vi "Initialize Motor.vi"() -> ()   [LabVIEW 2010]
panel:
  in  "Control units?":bool
  out "Enable\nReturn Value":i16
  out "Program\nReturn Value":i16
  out "Init\nReturn\nValue":i16
  out "Open\nDriver\nReturn\nValue":i16
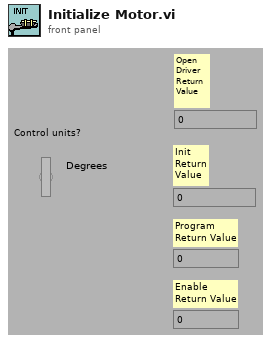
[diagram p1: front panel]
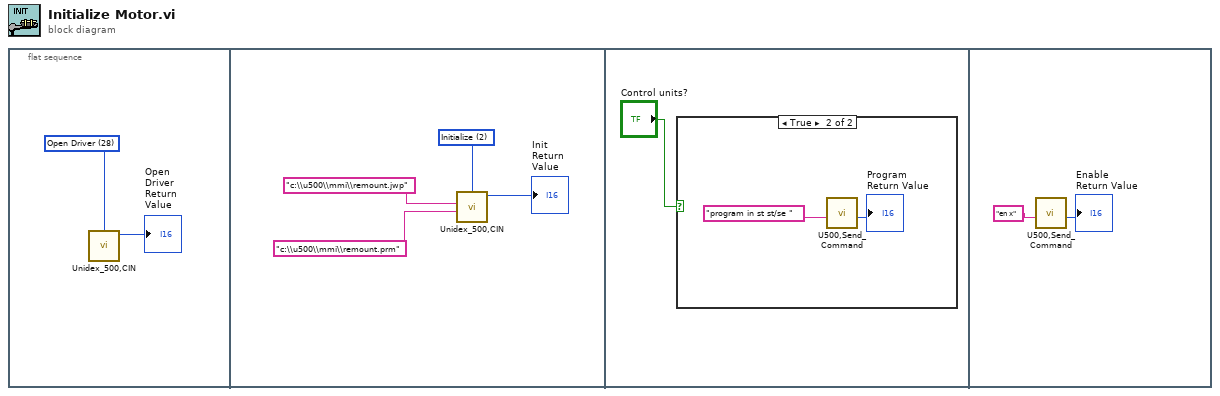
[diagram p0: block diagram]
diagram:
  n1 = flat-sequence {
    frame #0 {
      w2 = u16 28 items=["Send", "Retry", "Initialize", "Reset", "Abort", "CheckStatus", "Pause", "FaultAck", "Read_Variable", "Read_Position", "Read_Status", "Write_Param", "Read_Param", "Save_Param", "Write_Axcal", "Read_Axcal", "Save_Config", "Open_Param", "Open_Config", "Check_Initz", "Reset_Intr", "Set Velocity Timebase", "Enable Velocity Tracking", "Disable Velocity Tracking", "Read_Velocity", "Enable A/D Read", "Disable A/D Read", "Read A/D", "Open Driver", "Close Driver", "Get Error Message", "LoadCalFile", "LZR_Initialize", "LZRStop", "LZRCorrectionFactor"] ("Library Function")
      n2 = call "Unidex_500,CIN.VI"("Library Function"=w2) -> ("Return\nValue"=→"Open\nDriver\nReturn\nValue":i16)  [unwired: 5 in, 3 out]
    }
    frame #1 {
      w6 = u16 2 items=["Send", "Retry", "Initialize", "Reset", "Abort", "CheckStatus", "Pause", "FaultAck", "Read_Variable", "Read_Position", "Read_Status", "Write_Param", "Read_Param", "Save_Param", "Write_Axcal", "Read_Axcal", "Save_Config", "Open_Param", "Open_Config", "Check_Initz", "Reset_Intr", "Set Velocity Timebase", "Enable Velocity Tracking", "Disable Velocity Tracking", "Read_Velocity", "Enable A/D Read", "Disable A/D Read", "Read A/D", "Open Driver", "Close Driver", "Get Error Message", "LoadCalFile", "LZR_Initialize", "LZRStop", "LZRCorrectionFactor"] ("Library Function")
      n3 = call "Unidex_500,CIN.VI"("Library Function"=w6, "Firmware File Path"="c:\\u500\\mmi\\remount.jwp", "Parameter File Path"="c:\\u500\\mmi\\remount.prm") -> ("Return\nValue"=→"Init\nReturn\nValue":i16)  [unwired: 3 in, 3 out]
    }
    frame #2 {
      n4 = case shown="True" "Control units?" {
        frame False {
        }
        frame True {
          n5 = call "U500,Send_Command.vi"("Command String"="program in st st/se ") -> ("Return Value"=→"Program\nReturn Value":i16)  [unwired: 9 in, 1 out]
        }
      }
    }
    frame #3 {
      n6 = call "U500,Send_Command.vi"("Command String"="en x") -> ("Return Value"=→"Enable\nReturn Value":i16)  [unwired: 9 in, 1 out]
    }
  }
